vi "turn.vi"(0 "reference":refnum<class "Direction.lvclass">, 1 "angle":dbl format="%.2f", 5 "error in (no error)":errorcluster) -> (14 "reference out":refnum<class "Direction.lvclass">, 15 "turnedDirection":refnum<class "Direction.lvclass">, 19 "error out":errorcluster)   [LabVIEW 2012, in "Direction.lvclass"]
doc: "public Direction turn(double angle)"
uses:
  <resource>/Framework/Providers/Open_GDS/UML/Direction_class/Direction.lvclass
  <resource>/Framework/Providers/Open_GDS/UML/General/Point/Point Point2D.ctl
  <resource>/Framework/Providers/Open_GDS/UML/Direction_class/Direction.lvclass/Direction.ctl
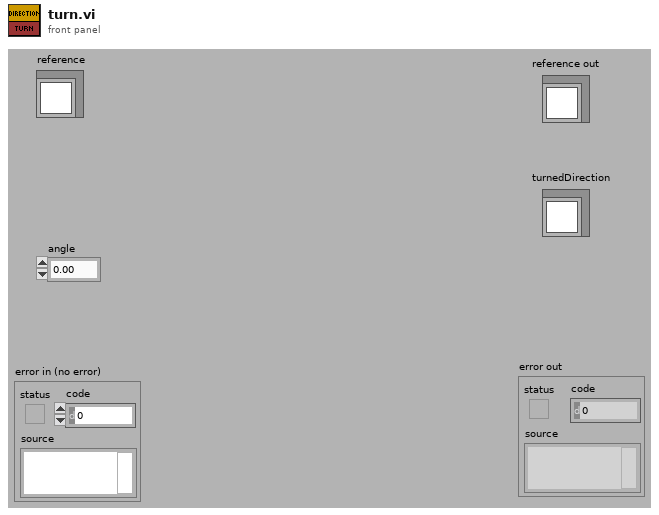
[diagram p1: front panel]
types:
  T1 = typedef "Point Point2D.ctl" = cluster{"x":dbl, "y":dbl}
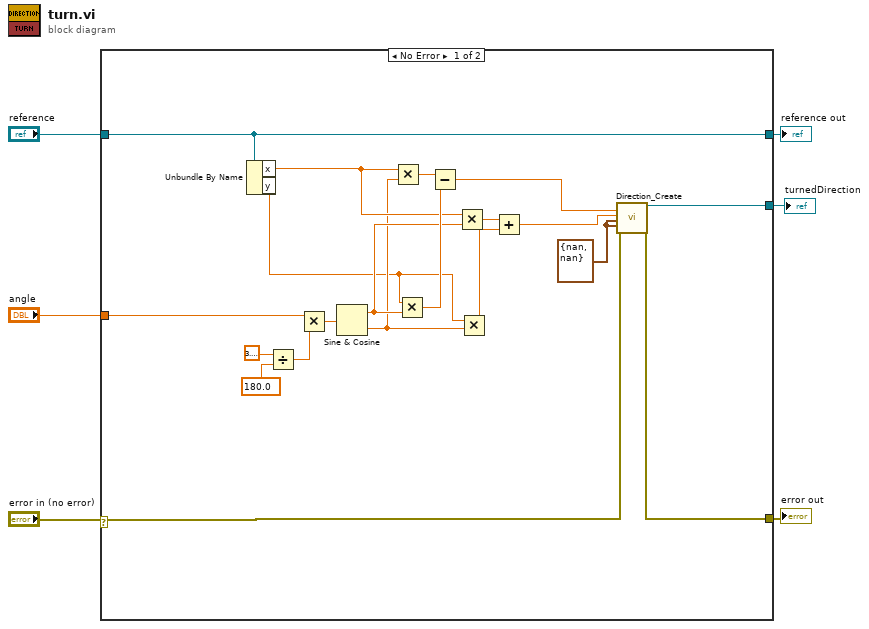
[diagram p0: block diagram]
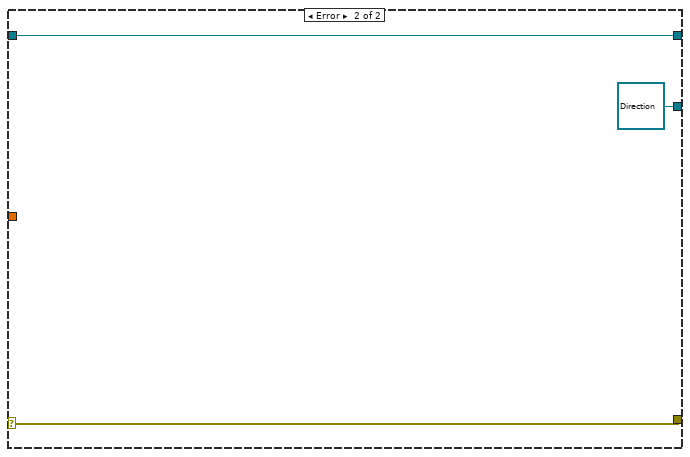
[diagram p2: hidden frame]
diagram:
  n1 = case shown="No Error" "error in (no error)" {
    selector: "error in (no error)" -> [w8 w28]
    tunnel: "reference" -> [w7 w29]
    tunnel: [w26 w28] -> w5
    tunnel: [w7 w29] -> w4
    tunnel: "angle" -> [w25 _]
    tunnel: [w24 refnum<class "Direction.lvclass"> refnum ("reference out")] -> w1
    frame No Error {
      w9 = T1 {"x"=nan, "y"=nan} ("p1")
      n2 = Unbundle By Name(w7) -> ("x"=w17:dbl, "y"=w14:dbl)
      n3 = Divide(x=3.141592653589793, y=180.0 ("x")) -> (x/y=w23:dbl)
      n4 = Multiply(x=w25, y=w23) -> (x*y=w22:dbl)
      n5 = Sine & Cosine(0:w22) -> (1:w16:dbl, 2:w15:dbl)
      n6 = Multiply(x=w17, y=w15) -> (x*y=w21:dbl)
      n7 = Multiply(x=w14, y=w16) -> (x*y=w20:dbl)
      n8 = Subtract(x=w21, y=w20) -> (x-y=w19:dbl)
      n9 = Multiply(x=w17, y=w16) -> (x*y=w18:dbl)
      n10 = Multiply(x=w14, y=w15) -> (x*y=w13:dbl)
      n11 = Add(x=w18, y=w13) -> (x+y=w12:dbl)
      n12 = call <resource>:"Direction_Create.vi"("dx"=w19, "dy"=w12, "p1"=w9, "p2"=w9, "error in (no error)"=w8) -> ("reference out"=w24:refnum<class "Direction.lvclass">, "error out"=w26:errorcluster)  [unwired: 13 in]
    }
    frame Error {
    }
  }
  "reference out" <- w4
  "error out" <- w5
  "turnedDirection" <- w1
